vi "Joystick Control Time Decay.vi"(2 "Delay (sec)":dbl=0.1, 4 "Value":dbl, 8 "Time Stamp":timestamp) -> (1 "Decayed Value":dbl)   [LabVIEW 2011]
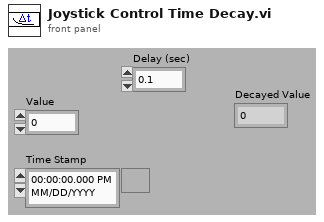
[diagram p1: front panel]
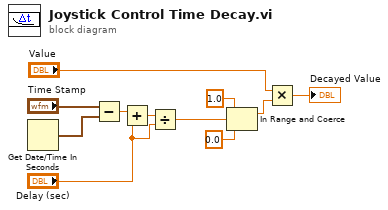
[diagram p0: block diagram]
diagram:
  n1 = Get Date/Time In Seconds() -> (seconds since 1Jan1904=w5:timestamp)
  n2 = Subtract(x="Time Stamp", y=w5) -> (x-y=w4:dbl)
  n3 = Add(x=w4, y="Delay (sec)") -> (x+y=w3:dbl)
  n4 = Divide(x=w3, y="Delay (sec)") -> (x/y=w1:dbl)
  n5 = In Range and Coerce(upper limit=1.0, x=w1, lower limit=0.0) -> (coerced(x)=w10:dbl)  [unwired: 1 out]
  n6 = Multiply(x="Value", y=w10) -> (x*y=→"Decayed Value":dbl)
